vi "Update System Status.vi"(8 "error in":errorcluster, 10 "System Status":T1, 11 "Base Software in":refnum<class "Main.lvclass">) -> (0 "error out":errorcluster, 3 "Base Software out":refnum<class "Main.lvclass">)   [LabVIEW 2023, in "Main.lvlib" / "Main.lvclass"]
doc: "This tool reads the system status and updates the state as needed\nThere is some complex state controls in here:\n\nIf we are sending a nominal status message -> we will update the state\nto the most recent \"Healthy State\" -> This assumes that we've transitioned\nfrom a warning or error state back to a healty state\n\nIf we are sending a warning message, update the current state to warning,\nbut retain the previous state so we can return to a healty state\n\nIf we are sending an erro message, update the current state to error,\nbut retain the previous state so we can return to a healty state\n\nAfter state data is updated, refresh the system state indicator"
uses:
  Project/Main.lvclass
  builds/Engine/Engine.lvlibp/Custom Controls/System Status.ctl
  Project/Main.lvclass/Main.ctl
  builds/Engine/Engine.lvlibp/Project/Engine.lvclass
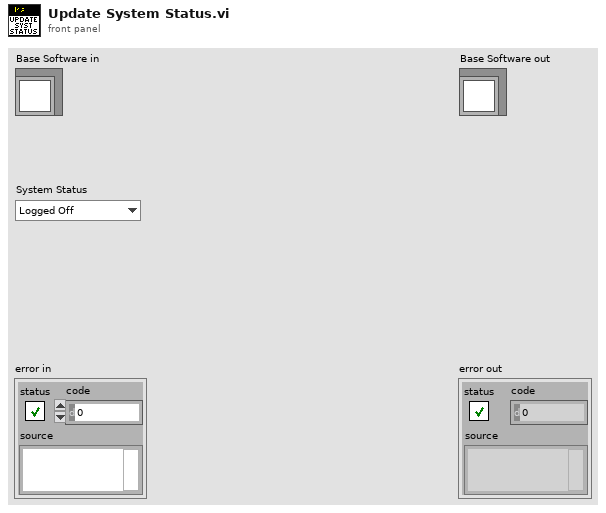
[diagram p1: front panel]
types:
  T1 = typedef "Engine.lvlibp/Engine.lvclass/System Status.ctl" = enum16{"Logged Off", "UUT_Info_Missing", "Idle", "Error", "Warning", "Loading", "Config", "Manual", "Automation", "Report_View", "Previous"}
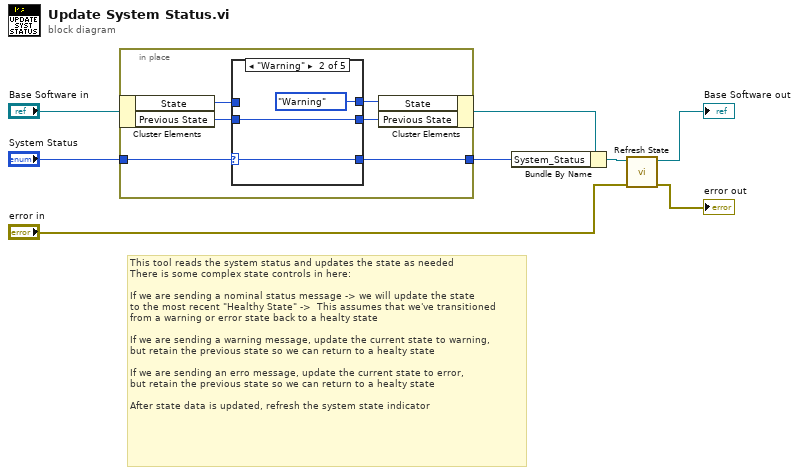
[diagram p0: block diagram]
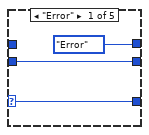
[diagram p2: hidden frame]
diagram:
  # "This tool reads the system status and updates the state as needed\nThere is some complex state controls in here:\n\nIf we are sending a nominal status message -> we will update the state\nto the most recent \"Healthy State\" ->  This assumes that we've transitioned\nfrom a warning or error state back to a healty state\n\nIf we are sending a warning message, update the current state to warning,\nbut retain the previous state so we can return to a healty state\n\nIf we are sending an erro message, update the current state to error,\nbut retain the previous state so we can return to a healty state\n\nAfter state data is updated, refresh the system state indicator"
  n1 = in-place {
    in-place-border: "System Status" -> [w14]
    in-place-border: [w9] -> w2
    n2 = in-place-cluster #1("Base Software in") -> ("State"=w13:T1, "Previous State"=w12:T1)
    n3 = case shown="\"Warning\"" w14 {
      selector: w14 -> [w16 w19 w21 w23 _]
      tunnel: w13 -> [_ _ _ _ _]
      tunnel: w12 -> [w17 w20 w22 _ w24]
      tunnel: [w17 w20 w22 w23 w24] -> w11
      tunnel: [System_Status."Error" ("Previous State") System_Status."Warning" ("Previous State") w22 w23 w24] -> w10
      tunnel: [w16 w19 w21 w23 w24] -> w9
      frame "Error" {
      }
      frame "Warning" {
      }
      frame "Logged Off" {
      }
      frame Default {
      }
      frame "Previous" {
      }
    }
    n4 = in-place-cluster #1("State"=w10, "Previous State"=w11) -> (w4:refnum<class "Main.lvclass">)
  }
  n5 = Bundle By Name(cluster=w4, "System_Status"=w2) -> (w8:refnum<class "Main.lvclass">)
  n6 = call "Refresh State.vi"("error in"="error in", "Base Software in"=w8) -> ("error out"=→"error out":errorcluster, "Base Software out"=→"Base Software out":refnum<class "Main.lvclass">)  [unwired: 8 in]
